vi "Name.vi"(8 "error in (no error)":errorcluster, 11 "Human in":refnum<class "Human.lvclass">) -> (0 "error out":errorcluster, 2 "Name":string, 3 "Human out":refnum<class "Human.lvclass">)   [LabVIEW 2020, in "Reversi.lvlib" / "Human.lvclass"]
uses:
  Human.lvclass
  Human.lvclass/Human.ctl
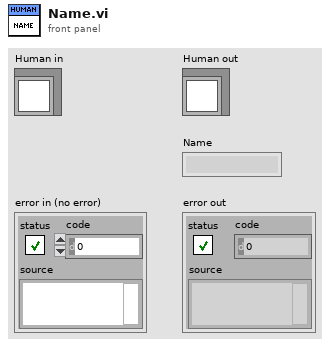
[diagram p1: front panel]
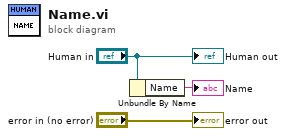
[diagram p0: block diagram]
diagram:
  n1 = Unbundle By Name("Human in") -> ("Name"=→"Name":string)
  "error out" <- "error in (no error)"
  "Human out" <- "Human in"
